vi "Read File prefix.vi"(8 "error in (no error)":errorcluster, 11 "Measure Controller in":refnum<class "Measure Controller.lvclass">) -> (0 "error out":errorcluster, 2 "File prefix":string="p", 3 "Measure Controller out":refnum<class "Measure Controller.lvclass">)   [LabVIEW 2015, in "Measure Controller.lvclass"]
uses:
  Measure Controller.lvclass
  Measure Controller.lvclass/Measure Controller.ctl
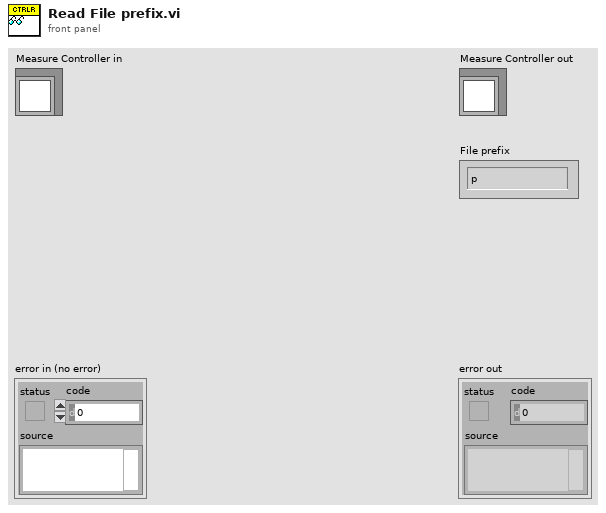
[diagram p1: front panel]
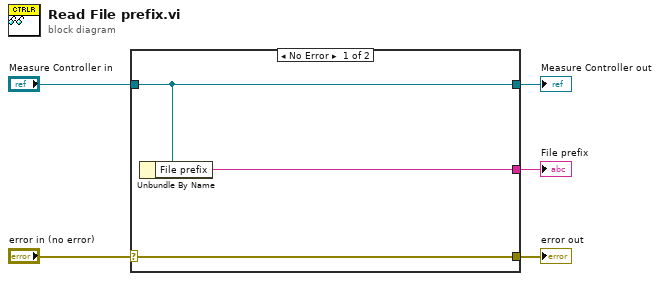
[diagram p0: block diagram]
diagram:
  n1 = case shown="No Error" "error in (no error)" {
    selector: "error in (no error)" -> [w8 w9]
    tunnel: [w8 w9] -> w4
    tunnel: [w7 w10] -> w2
    tunnel: "Measure Controller in" -> [w7 w10]
    tunnel: [w6 _] -> w1
    frame No Error {
      n2 = Unbundle By Name(w7) -> ("File prefix"=w6:string)
    }
    frame Error {
    }
  }
  "error out" <- w4
  "Measure Controller out" <- w2
  "File prefix" <- w1
